vi "Intake_Test.vi"(11 "Joystick_In":T1) -> ()   [LabVIEW 2019]
uses:
  Utility_VIs/Joystick_Controls.ctl
  Subsystems/Intake/Intake_Cluster.ctl
  Subsystems/Intake/Intake_States.ctl
  Globals/Intake_Globals.vi
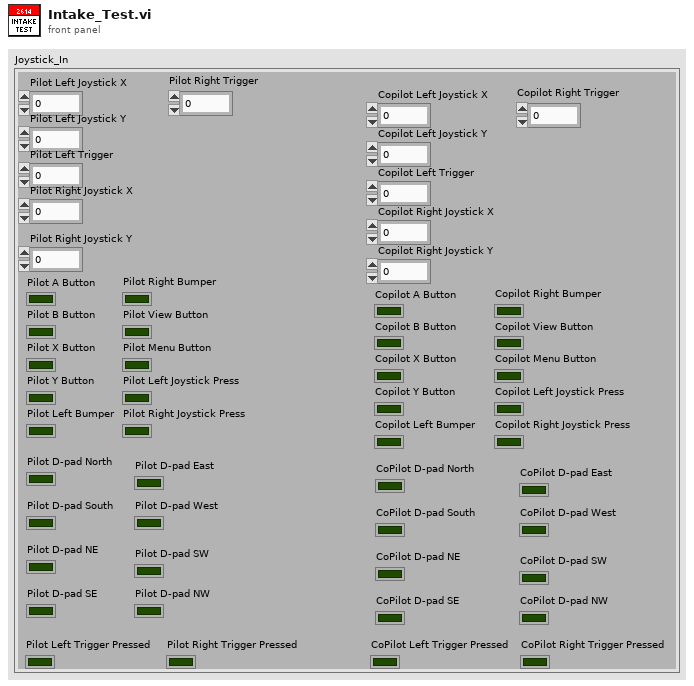
[diagram p1: front panel]
types:
  T1 = typedef "Joystick_Controls.ctl" = cluster{"Pilot Left Joystick X":dbl, "Pilot Left Joystick Y":dbl, "Pilot A Button":bool, "Pilot B Button":bool, "Pilot X Button":bool, "Pilot Y Button":bool, "Pilot Left Bumper":bool, "Pilot Right Bumper":bool, "Pilot View Button":bool, "Pilot Menu Button":bool, "Pilot Left Joystick Press":bool, "Pilot Right Joystick Press":bool, "Pilot Left Trigger":dbl, "Pilot Right Joystick X":dbl, "Pilot Right Joystick Y":dbl, "Pilot Right Trigger":dbl, "Copilot Left Joystick X":dbl, "Copilot Left Joystick Y":dbl, "Copilot A Button":bool, "Copilot B Button":bool, "Copilot X Button":bool, "Copilot Y Button":bool, "Copilot Left Bumper":bool, "Copilot Right Bumper":bool, "Copilot View Button":bool, "Copilot Menu Button":bool, "Copilot Left Joystick Press":bool, "Copilot Right Joystick Press":bool, "Copilot Left Trigger":dbl, "Copilot Right Joystick X":dbl, "Copilot Right Joystick Y":dbl, "Copilot Right Trigger":dbl, "Pilot D-pad North":bool, "Pilot D-pad South":bool, "Pilot D-pad East":bool, "Pilot D-pad West":bool, "Pilot D-pad NE ":bool, "Pilot D-pad SE":bool, "Pilot D-pad SW":bool, "Pilot D-pad NW":bool, "CoPilot D-pad North":bool, "CoPilot D-pad South":bool, "CoPilot D-pad East":bool, "CoPilot D-pad West":bool, "CoPilot D-pad NE":bool, "CoPilot D-pad SE":bool, "CoPilot D-pad SW":bool, "CoPilot D-pad NW":bool, "Pilot Left Trigger Pressed":bool, "Pilot Right Trigger Pressed":bool, "CoPilot Left Trigger Pressed":bool, "CoPilot Right Trigger Pressed":bool}
  T2 = typedef "Intake_Cluster.ctl" = cluster{"Control_State":T3, "Intake":bool, "Intake_Extended":bool, "Intake_Throttle":dbl, "Outtake":bool}
  T3 = typedef "Intake_States.ctl" = enum16{"Manual_Control", "Compliant_Intake"}
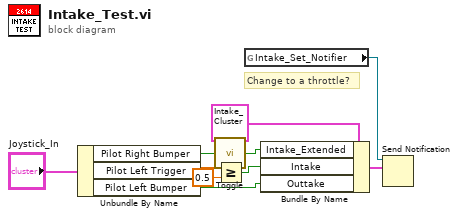
[diagram p0: block diagram]
diagram:
  # "Change to a throttle?"
  n1 = Unbundle By Name("Joystick_In") -> ("Pilot Right Bumper"=w5:bool, "Pilot Left Trigger"=w2:dbl, "Pilot Left Bumper"=w6:bool)
  n2 = call "Toggle.vi"("Boolean"=w5) -> ("Boolean Out"=w4:bool)
  n3 = Greater Or Equal?(x=w2, y=0.5) -> (x >= y?=w3:bool)
  n4 = global read "Intake_Globals.vi" "Intake_Set_Notifier"() -> (w9:refnum<notifier>)
  n5 = Bundle By Name(cluster=T2 {"Control_State"=enum."Manual_Control", "Intake"=FALSE, "Intake_Extended"=FALSE, "Intake_Throttle"=0.0, "Outtake"=FALSE} ("notification"), "Intake_Extended"=w4, "Intake"=w3, "Outtake"=w6) -> (w7:T2)
  n6 = Send Notification(notification=w7, notifier=w9) -> ()  [unwired: 1 in, 2 out]
